vi "Init.vi"(8 "error in (no error)":errorcluster, 10 "GameName":string, 11 "Highscore in":refnum<class "Highscore.lvclass">) -> (0 "error out":errorcluster, 3 "Highscore out":refnum<class "Highscore.lvclass">)   [LabVIEW 2019, in "RT_Game.lvlib" / "Highscore.lvclass"]
uses:
  Highscore.lvclass
  HighscoreEntry.ctl
  Highscore.lvclass/Highscore.ctl
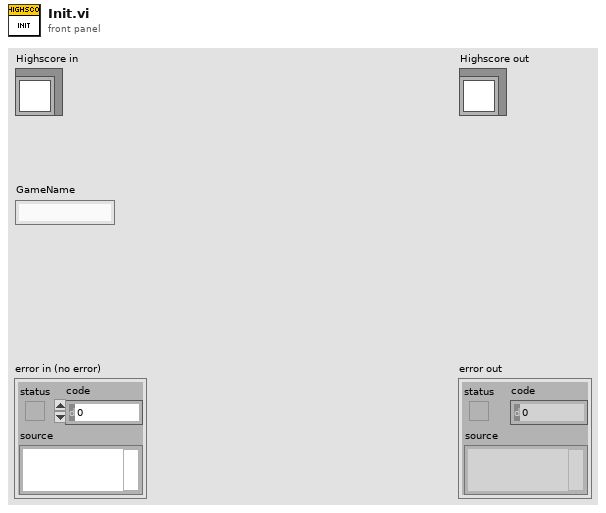
[diagram p1: front panel]
types:
  T1 = typedef "RT_Game.lvlib/Highscore.lvclass/HighscoreEntry.ctl" = cluster{"Name":string, "Score":dbl}
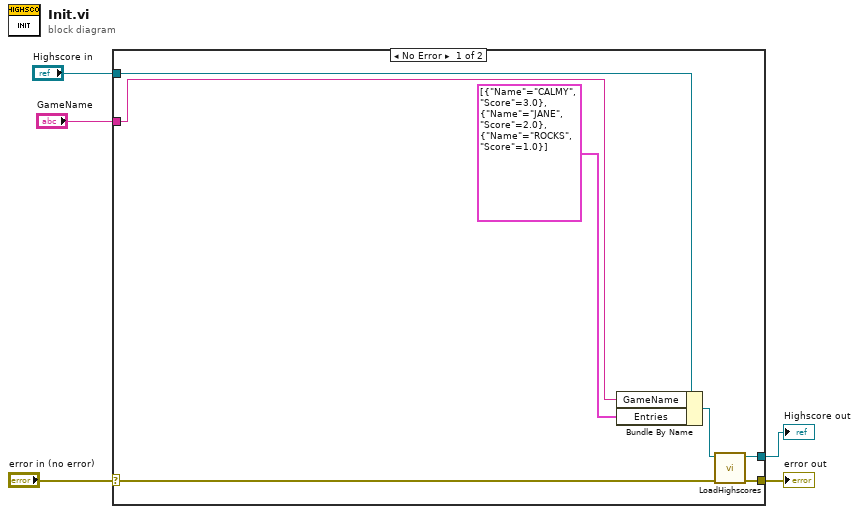
[diagram p0: block diagram]
diagram:
  n1 = case shown="No Error" "error in (no error)" {
    selector: "error in (no error)" -> [w11 w14]
    tunnel: [w9 w14] -> w4
    tunnel: [w7 w13] -> w2
    tunnel: "Highscore in" -> [w12 w13]
    tunnel: "GameName" -> [w10 _]
    frame No Error {
      n2 = Bundle By Name(cluster=w12, "GameName"=w10, "Entries"=T1[] [{"Name"="CALMY", "Score"=3.0}, {"Name"="JANE", "Score"=2.0}, {"Name"="ROCKS", "Score"=1.0}] ("t")) -> (w8:refnum<class "Highscore.lvclass">)
      n3 = call "LoadHighscores.vi"("error in (no error)"=w11, "Highscore in"=w8) -> ("error out"=w9:errorcluster, "Highscore out"=w7:refnum<class "Highscore.lvclass">)  [unwired: 8 in]
    }
    frame Error {
    }
  }
  "error out" <- w4
  "Highscore out" <- w2
